vi "Keithley 6487 Exit.vi"(1 "error in (no error)":errorcluster, 2 "VISA resource name":refnum<visa-resource-name>) -> (0 "error out":errorcluster)   [LabVIEW 2018]
panel:
  in  "Exit Configuration":string=":SOUR:VOLT 0;:SOUR:VOLT:STAT 0;:SYST:LOC"
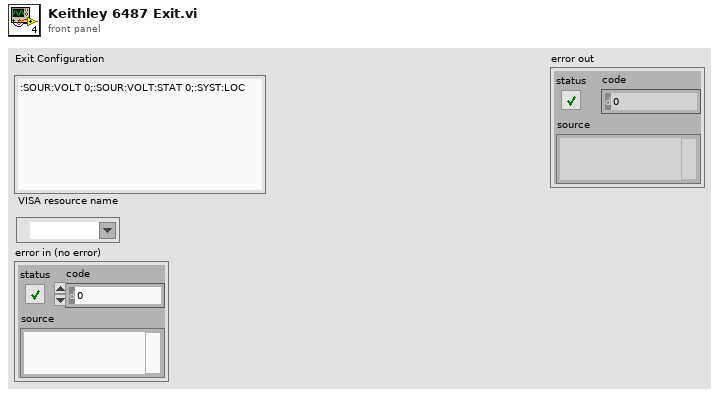
[diagram p1: front panel]
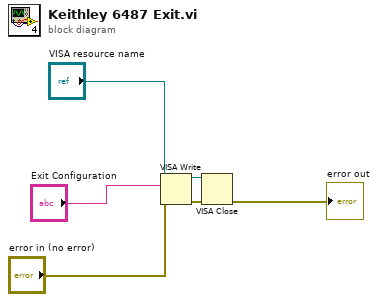
[diagram p0: block diagram]
diagram:
  n1 = VISA Write(VISA resource name="VISA resource name", write buffer="Exit Configuration", error in (no error)="error in (no error)") -> (VISA resource name out=w4:refnum<visa-resource-name>, error out=w5:errorcluster)  [unwired: 1 out]
  n2 = VISA Close(VISA resource name=w4, error in (no error)=w5) -> (error out=→"error out":errorcluster)
